vi "UMB_Arbiter.vi"(11 "Behavior Data":T1=[{"Goodness"=[0, 0, 0, 0, 0, 0, 0, 0, 0, 0, 0, 0, 0, 0, 0], "Velocity"=[0, 0, 0, 0, 0, 0, 0, 0, 0, 0, 0, 0, 0, 0, 0], "Weight"=0}]) -> (1 "prop":i8, 2 "rudder":i32)   [LabVIEW 2012]
uses:
  NINJA Code/Tugboat/Robo_Programs/behaviorData_t.ctl
  NINJA Code/Tugboat/Robo_Programs/behaviorOutput_t.ctl
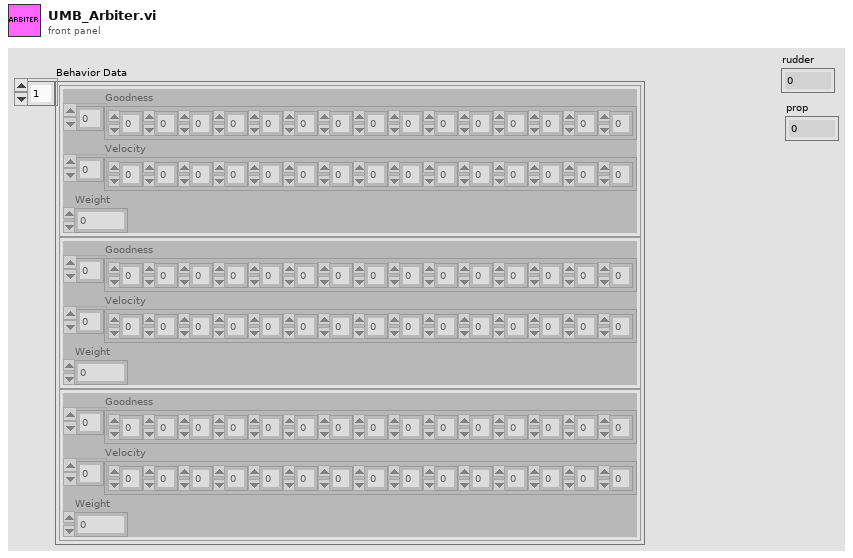
[diagram p1: front panel]
types:
  T1 = typedef "behaviorData_t.ctl" = T2[]
  T2 = typedef "behaviorOutput_t.ctl" = cluster{"Goodness":i8[], "Velocity":i8[], "Weight":i8}
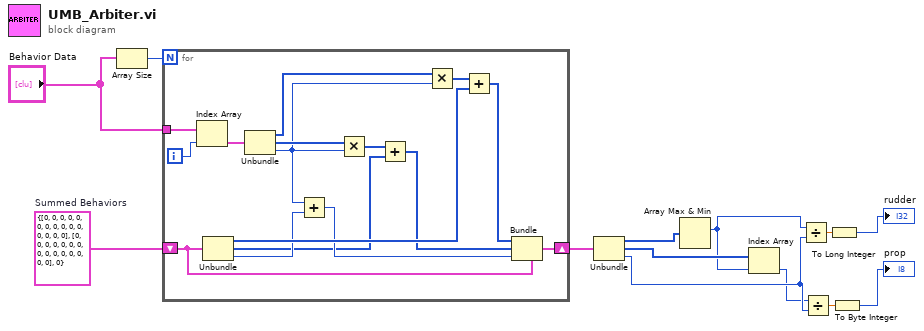
[diagram p0: block diagram]
diagram:
  w12 = T2 {"Goodness"=[0, 0, 0, 0, 0, 0, 0, 0, 0, 0, 0, 0, 0, 0, 0], "Velocity"=[0, 0, 0, 0, 0, 0, 0, 0, 0, 0, 0, 0, 0, 0, 0], "Weight"=0}  # Summed Behaviors
  n1 = Array Size(array="Behavior Data") -> (size(s)=w13:i32)
  n2 = for {
    N: w13 -> [_]
    shift-right: [w24] -> w10
    shift-left: w12 -> [w25]
    tunnel: "Behavior Data" -> [w28]
    i -> [w29]
    n3 = Index Array(array=w28, index=w29) -> (element=w27:T2)
    n4 = Unbundle(w25) -> ("Goodness"=w22:i8[], "Velocity"=w15:i8[], "Weight"=w20:i8)
    n5 = Unbundle(w27) -> ("Goodness"=w26:i8[], "Velocity"=w18:i8[], "Weight"=w17:i8)
    n6 = Add(x=w17, y=w20) -> (x+y=w19:i8)
    n7 = Multiply(x=w18, y=w17) -> (x*y=w16:i8[])
    n8 = Add(x=w16, y=w15) -> (x+y=w14:i8[])
    n9 = Multiply(x=w26, y=w17) -> (x*y=w23:i8[])
    n10 = Add(x=w23, y=w22) -> (x+y=w21:i8[])
    n11 = Bundle(cluster=w25, "Goodness"=w21, "Velocity"=w14, "Weight"=w19) -> (w24:T2)
  }
  n12 = Unbundle(w10) -> ("Goodness"=w9:i8[], "Velocity"=w8:i8[], "Weight"=w7:i8)
  n13 = Array Max & Min(array=w9) -> (max index (indices)=w6:i32)  [unwired: 3 out]
  n14 = Index Array(array=w8, index=w6) -> (element=w4:i8)
  n15 = Divide(x=w6, y=w7) -> (x/y=w5:dbl)
  n16 = Divide(x=w4, y=w7) -> (x/y=w3:dbl)
  n17 = To Long Integer(number=w5) -> (32bit integer=→"rudder":i32)
  n18 = To Byte Integer(number=w3) -> (8bit integer=→"prop":i8)
